vi "File Write Matrix.vi"(0 "file path (dialog if empty)":path, 5 "Matrix":dbl[][](array[numeric]), 7 "Row Names":string[](array[string]), 9 "Column Names":string[](array[string]), 11 "error in (no error)":errorcluster, 12 "Beam Energy (MeV)":dbl) -> (15 "error out":errorcluster)   [LabVIEW 2011, in "File VIs.lvlib"]
doc: "Writes a 2D, double-precision array of numbers into a \"Response Matrix\" or \"Correction Matrix\" text file.\n\nFile format:\nFirst row: Beam Energy (MeV):<TAB>[Beam Energy Value for which the matrix was measured/calculated]\nSecond row*: Column names (Corrector names, for Response Matrix; BPM names, for Correction Matrix)\nAll other rows:\n Column 1: BPM names\n All other columns: Matrix value (mm/A, for Response Matrix; A/mm, for Correction Matrix)\nColumn separator: <TAB> character\n\n* The second row must begin with a <TAB> character\n\nEx.:\nBeam Energy (MeV):<TAB>1370\n<TAB>ACH01B<TAB>ACH02\nAMP01BH<TAB>5.10765701<TAB>-1.50432895\nAMP02AH<TAB>-0.41130998<TAB>0.95389896"
uses:
  File VIs.lvlib
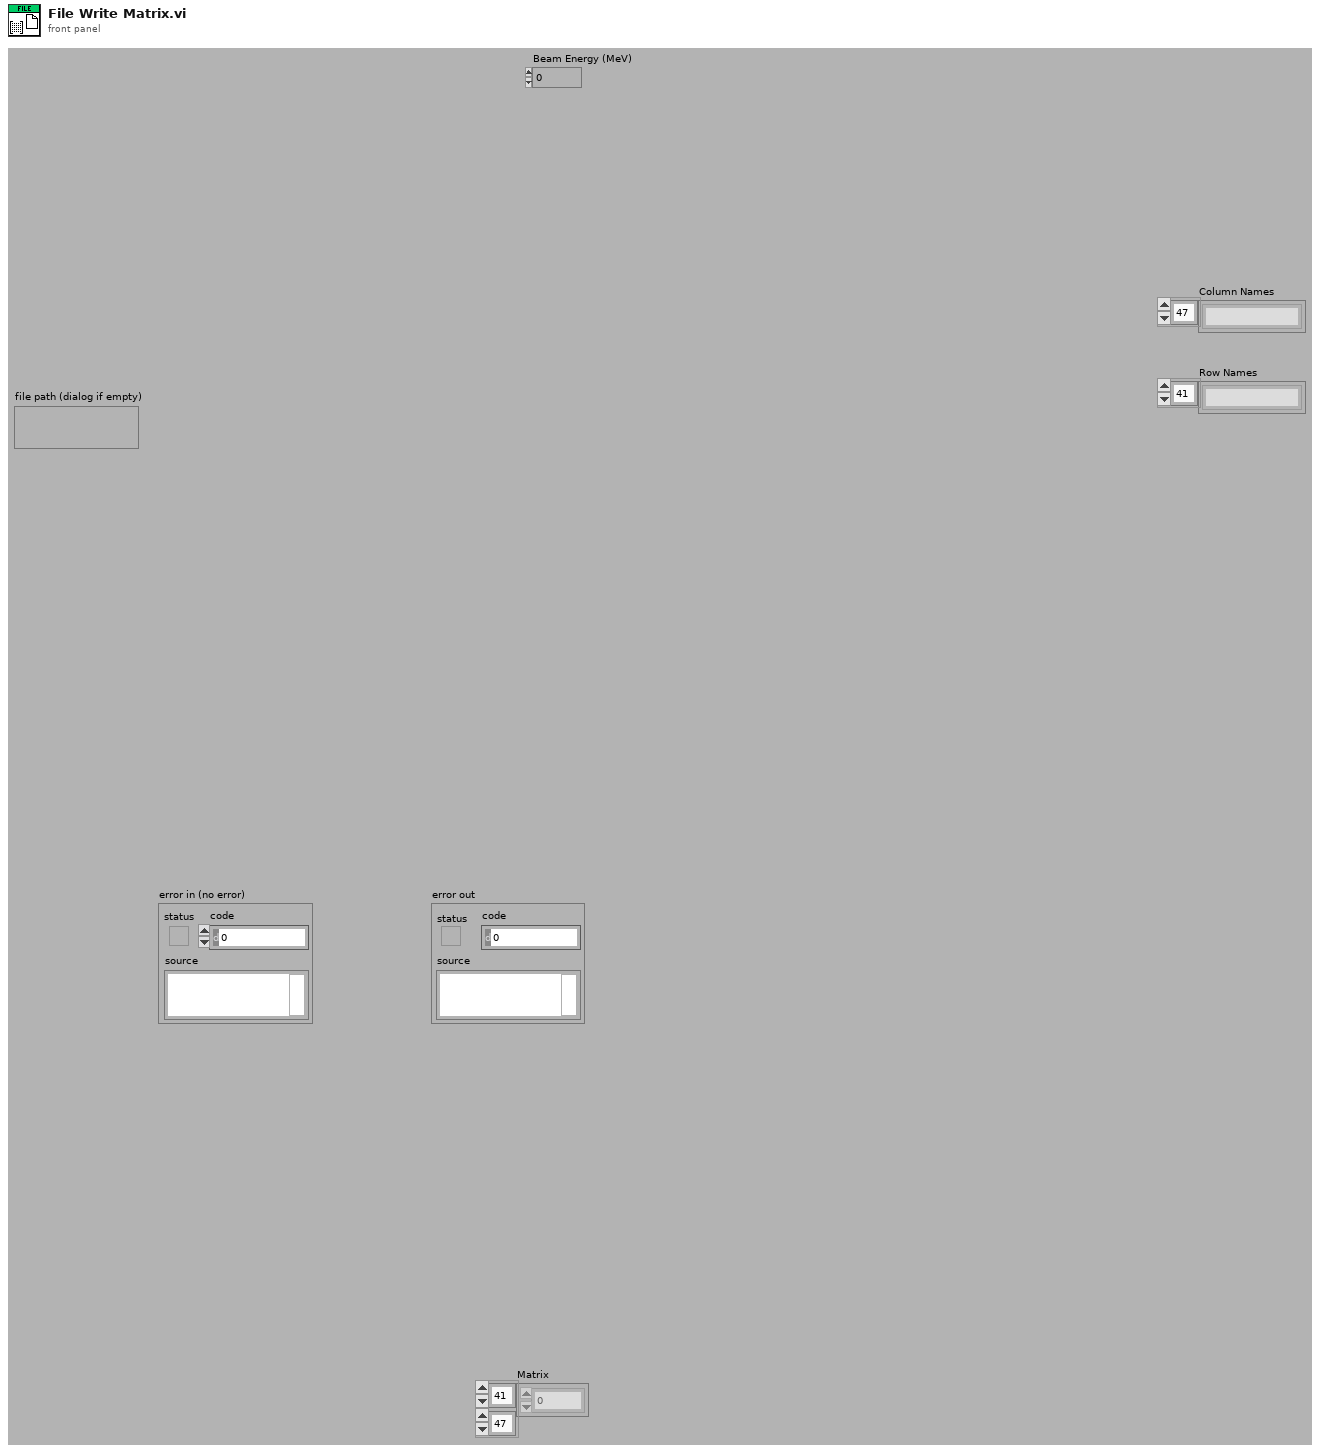
[diagram p1: front panel]
types:
  T1 = enum16{"open", "replace", "create", "open or create", "replace or create", "replace or create with confirmation"}
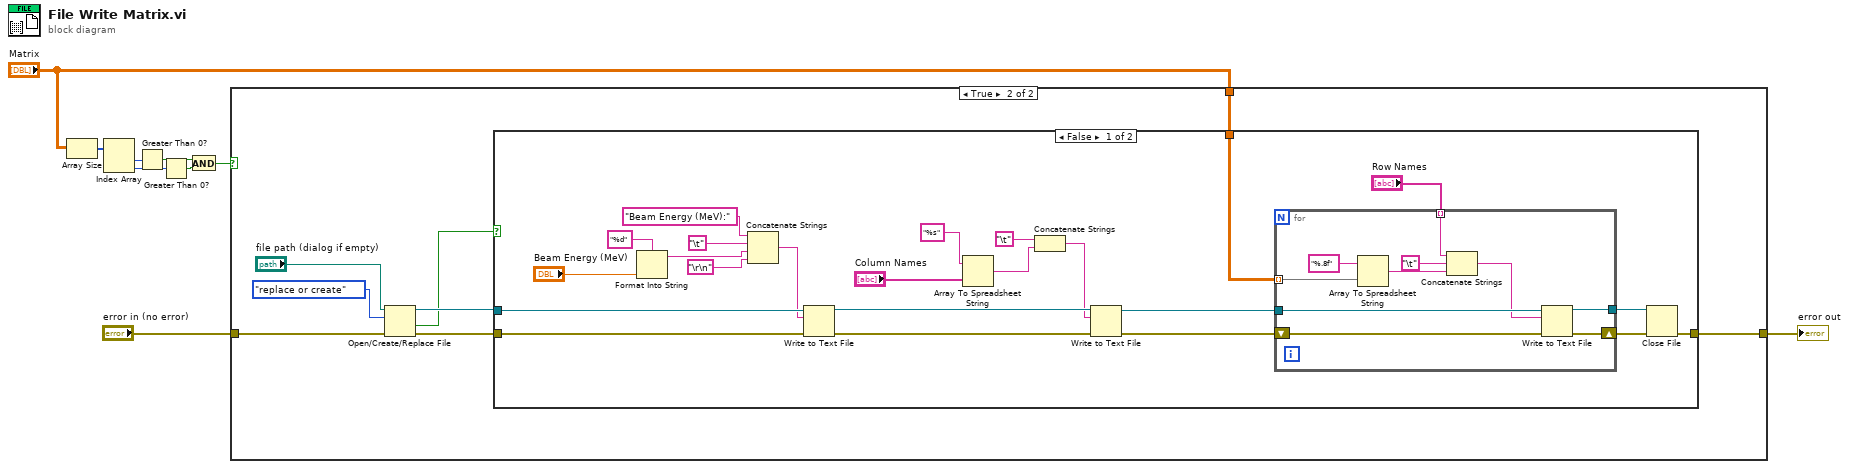
[diagram p0: block diagram]
diagram:
  n1 = Array Size(array="Matrix") -> (size(s)=w6:i32[])
  n2 = Index Array(array=w6) -> (element #1=w5:i32, element #2=w4:i32)  [unwired: 2 in]
  n3 = Greater Than 0?(x=w5) -> (x > 0?=w3:bool)
  n4 = Greater Than 0?(x=w4) -> (x > 0?=w2:bool)
  n5 = And(x=w3, y=w2) -> (x .and. y?=w1:bool)
  n6 = case shown="True" w1 {
    tunnel: [w10 w18] -> w9
    tunnel: "error in (no error)" -> [w10 w12]
    tunnel: "Matrix" -> [_ w11]
    frame False {
    }
    frame True {
      n7 = Open/Create/Replace File(file path (use dialog)="file path (dialog if empty)", error in=w12, operation (0:open)=T1."replace or create") -> (refnum out=w15:refnum<file>, cancelled=w13:bool, error out=w14:errorcluster)  [unwired: 3 in]
      n8 = case shown="False" w13 {
        tunnel: [w41 w52] -> w18
        tunnel: w15 -> [w35 _]
        tunnel: w14 -> [w38 w52]
        tunnel: w11 -> [w19 _]
        frame False {
          n9 = Format Into String(format string="%d", "Beam Energy (MeV)") -> (resulting string=w30:string)  [unwired: 2 in, 1 out]
          n10 = Concatenate Strings("Beam Energy (MeV):" ("format (%.3f)"), "\t", w30, "\r\n") -> (w26:string)
          n11 = Write to Text File(file (use dialog)=w35, text=w26, error in=w38) -> (refnum out=w34:refnum<file>, error out=w37:errorcluster)  [unwired: 1 in, 1 out]
          n12 = Array To Spreadsheet String(array="Column Names", 3:"%s" ("format string")) -> (spreadsheet string=w23:string)  [unwired: 1 in]
          n13 = Concatenate Strings("\t", w23) -> (w22:string)
          n14 = Write to Text File(file (use dialog)=w34, text=w22, error in=w37) -> (refnum out=w33:refnum<file>, error out=w36:errorcluster)  [unwired: 1 in, 1 out]
          n15 = for {
            tunnel: w19 -> [w50] mode=indexing
            shift-right: [w45] -> w40
            shift-left: w36 -> [w46]
            tunnel: "Row Names" -> [w47] mode=indexing
            tunnel: w33 -> [w44]
            tunnel: [w43] -> w39
            n16 = Array To Spreadsheet String(array=w50, 3:"%.8f" ("format (%.3f)")) -> (spreadsheet string=w48:string)  [unwired: 1 in]
            n17 = Concatenate Strings(w47, "\t", w48) -> (w42:string)
            n18 = Write to Text File(file (use dialog)=w44, text=w42, error in=w46) -> (refnum out=w43:refnum<file>, error out=w45:errorcluster)  [unwired: 1 in, 1 out]
          }
          n19 = Close File(refnum=w39, error in=w40) -> (error out=w41:errorcluster)  [unwired: 1 out]
        }
        frame True {
        }
      }
    }
  }
  "error out" <- w9
